vi "ReadWrite.EngineData.vi"(8 "error in":errorcluster, 11 "ReadWrite in":refnum<class "ReadWrite.lvclass">) -> (0 "error out":errorcluster, 3 "ReadWrite out":refnum<class "ReadWrite.lvclass">)   [LabVIEW 2024, in "VS Plugin Inline Async API.lvlib" / "ReadWrite.lvclass"]
uses:
  ReadWrite.lvclass
  ReadWrite.lvclass/ReadWrite.ctl
  VS Engine Interface/VS Engine Interface.lvclass
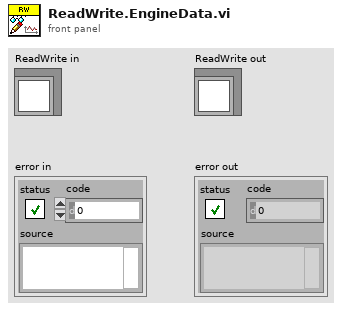
[diagram p1: front panel]
types:
  T1 = typedef "Custom Device API.lvlib/Data Reference.ctl" = i32
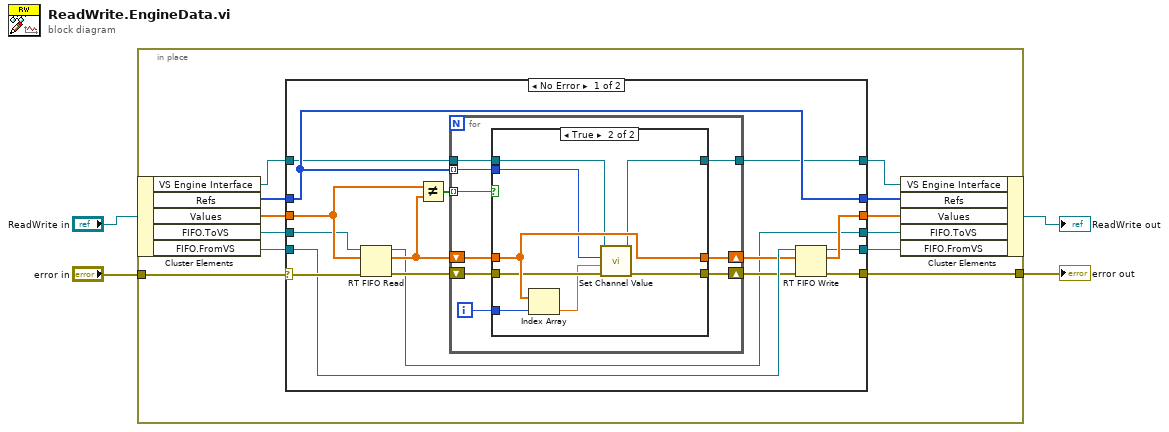
[diagram p0: block diagram]
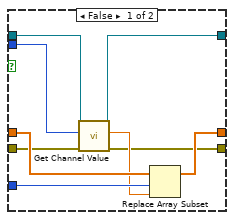
[diagram p2: hidden frame]
diagram:
  n1 = in-place {
    in-place-border: [w16] -> w1
    in-place-border: "error in" -> [w11]
    n2 = in-place-cluster #1("ReadWrite in") -> ("VS Engine Interface"=w6:refnum<class "VS Engine Interface.lvclass">, "Refs"=w15:T1[], "Values"=w14:dbl[], "FIFO.ToVS"=w9:refnum<k33>, "FIFO.FromVS"=w10:refnum<k33>)
    n3 = case shown="No Error" w11 {
      selector: w11 -> [w29 w63]
      tunnel: [w31 w63] -> w16
      tunnel: [w22 w62] -> w13
      tunnel: w15 -> [w21 w61]
      tunnel: w14 -> [w28 w62]
      tunnel: [w21 w61] -> w12
      tunnel: w9 -> [w26 w60]
      tunnel: w10 -> [w25 w59]
      tunnel: [w19 w60] -> w8
      tunnel: [w20 w59] -> w7
      tunnel: w6 -> [w18 w58]
      tunnel: [w17 w58] -> w5
      frame No Error {
        n4 = RT FIFO Read(0:w26, 1:w28, 3:w29) -> (8:w19:refnum<k33>, 9:w27:dbl[], 11:w30:errorcluster)  [unwired: 1 in, 2 out]
        n5 = Not Equal?(x=w28, y=w27) -> (x != y?=w24:bool[])
        n6 = for {
          shift-right: [w40] -> w23
          shift-left: w30 -> [w39]
          tunnel: w24 -> [w36] mode=indexing
          tunnel: w21 -> [w37] mode=indexing
          shift-right: [w34] -> w22
          shift-left: w27 -> [w38]
          tunnel: w18 -> [w33]
          tunnel: [w32] -> w17
          i -> [w35]
          n7 = case shown="True" w36 {
            tunnel: w38 -> [w48 w56]
            tunnel: [w41 w54] -> w40
            tunnel: w39 -> [w42 w55]
            tunnel: w37 -> [w45 w52]
            tunnel: w35 -> [w49 w57]
            tunnel: [w47 w56] -> w34
            tunnel: w33 -> [w46 w51]
            tunnel: [w43 w50] -> w32
            frame False {
              n8 = call-dynamic "Get Channel Value.vi"("error in"=w42, "Data Reference in"=w45, "VS Engine Interface in"=w46) -> ("error out"=w41:errorcluster, "Value"=w44:dbl, "VS Engine Interface out"=w43:refnum<class "VS Engine Interface.lvclass">)  [unwired: 6 in]
              n9 = Replace Array Subset(array=w48, new element=w44, index=w49) -> (w47:dbl[])
            }
            frame True {
              n10 = Index Array(array=w56, index=w57) -> (element=w53:dbl)
              n11 = call-dynamic "Set Channel Value.vi"("error in"=w55, "Value"=w53, "Data Reference in"=w52, "VS Engine Interface in"=w51) -> ("error out"=w54:errorcluster, "VS Engine Interface out"=w50:refnum<class "VS Engine Interface.lvclass">)  [unwired: 6 in]
            }
          }
        }
        n12 = RT FIFO Write(0:w25, 1:w22, 3:w23) -> (8:w20:refnum<k33>, 11:w31:errorcluster)  [unwired: 2 in, 2 out]
      }
      frame Error {
      }
    }
    n13 = in-place-cluster #1("VS Engine Interface"=w5, "Refs"=w12, "Values"=w13, "FIFO.ToVS"=w8, "FIFO.FromVS"=w7) -> (→"ReadWrite out":refnum<class "ReadWrite.lvclass">)
  }
  "error out" <- w1
